vi "Dig.vi"(8 "Error In":errorcluster) -> (0 "Error Out":errorcluster)   [LabVIEW 2017, in "Tests.lvlib"]
uses:
  Tests.lvlib
  src/Toolkit VIs/Toolkit.lvlib
  <vilib>/addons/_JKI Toolkits/Caraya/classes/Assert/Assert.lvclass
  <vilib>/addons/_JKI Toolkits/Caraya/classes/Test/Test.lvclass
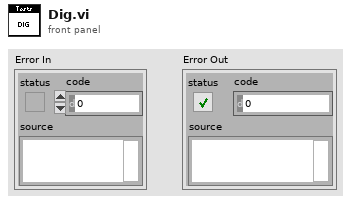
[diagram p1: front panel]
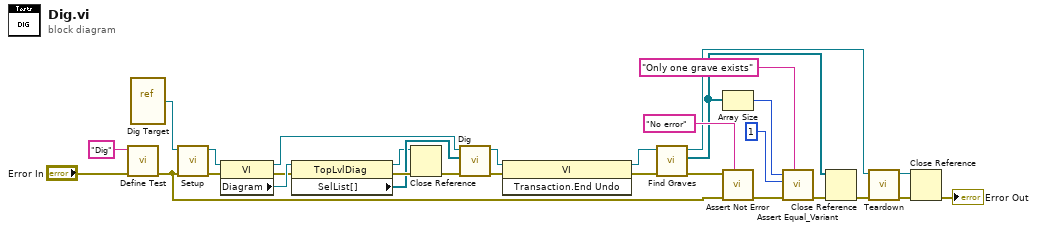
[diagram p0: block diagram]
diagram:
  n1 = call <vilib>:"Define Test.vi"("error in (no error)"="Error In", "Label (VI Title)"="Dig") -> ("error out"=w5:errorcluster)  [unwired: 9 in]
  n2 = vi-ref "Dig Target.vi"() -> (w27:refnum<vi>)
  n3 = call "Setup.vi"("Error In"=w5, "VI In"=w27) -> ("Error Out"=w4:errorcluster, "VI Out"=w6:refnum<vi>)  [unwired: 8 in]
  n4 = property class="VI"(reference=w6, error in=w4) -> (reference out=w26:refnum<vi>, error out=w29:errorcluster, "Diagram"=w30:refnum<vi>)
  n5 = property class="TopLvlDiag"(reference=w30, error in=w29) -> (reference out=w14:refnum<vi>, error out=w28:errorcluster, "SelList[]"=w25:refnum<vi>[])
  n6 = Close Reference(reference=w14, error in (no error)=w28) -> (error out=w15:errorcluster)
  n7 = call "Dig.vi"("Error In"=w15, "Selection List[]"=w25, "VI In"=w26) -> ("Error Out"=w23:errorcluster, "VI Out"=w24:refnum<vi>)  [unwired: 7 in]
  n8 = invoke class="VI" method="Transaction.End Undo"(reference=w24, error in=w23) -> (reference out=w21:refnum<vi>, error out=w22:errorcluster)  [unwired: 1 in, 1 out]
  n9 = call "Find Graves.vi"("Error In"=w22, "VI In"=w21) -> ("Error Out"=w16:errorcluster, "Graves"=w7:refnum<vi>[], "VI Out"=w9:refnum<vi>)  [unwired: 7 in]
  n10 = Array Size(array=w7) -> (size(s)=w13:i32)
  n11 = call <vilib>:"Assert Not Error.vi"("Label"="No error", "error in (no error)"=w5, "Not Error?"=w16) -> ("error out"=w18:errorcluster)  [unwired: 8 in]
  n12 = call <vilib>:"Assert Equal_Variant.vi"("Label"="Only one grave exists", "error in (no error)"=w18, "Y"=1 ("size(s)"), "X"=w13) -> ("error out"=w10:errorcluster)  [unwired: 7 in]
  n13 = Close Reference(reference=w7, error in (no error)=w10) -> (error out=w2:errorcluster)
  n14 = call "Teardown.vi"("Error In"=w2, "VI In"=w9) -> ("Error Out"=w1:errorcluster, "VI Out"=w3:refnum<vi>)  [unwired: 8 in]
  n15 = Close Reference(reference=w3, error in (no error)=w1) -> (error out=→"Error Out":errorcluster)
